vi "设置实验目录.vi"() -> ()   [LabVIEW 2013]
panel:
  in  "stop":bool
  in  "实验文件夹":path
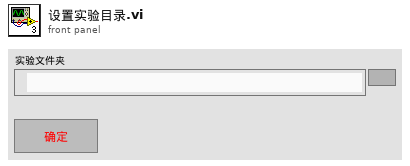
[diagram p1: front panel]
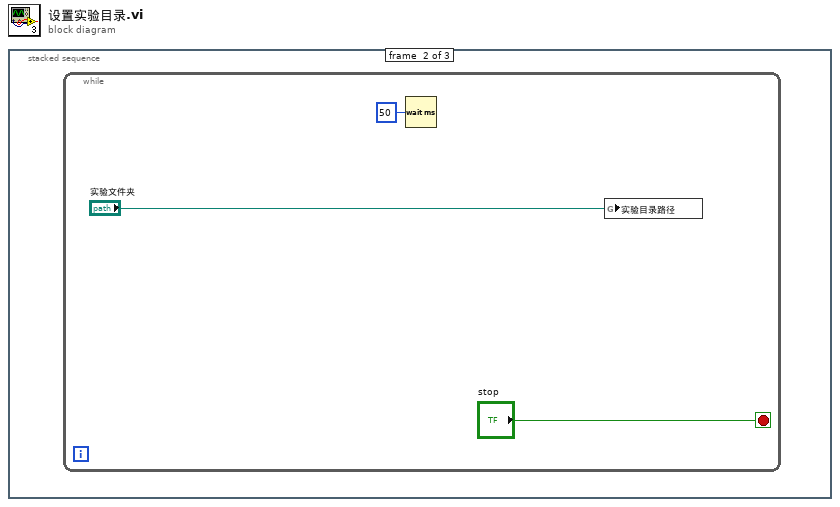
[diagram p0: block diagram]
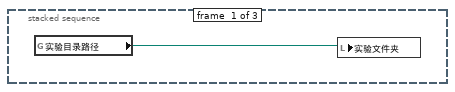
[diagram p2: hidden frame]
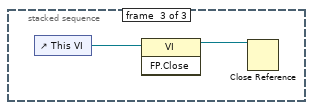
[diagram p3: hidden frame]
diagram:
  n1 = stacked-sequence {
    frame #0 {
      n2 = global read "实验目录路径.vi" "实验目录路径"() -> (w1:path)
      n3 = local write "实验文件夹"(w1) -> ()
    }
    frame #1 {
      n4 = while {
        stop <- "stop" stop-if-true
        n5 = Wait (ms)(milliseconds to wait=u32 50) -> ()  [unwired: 1 out]
        n6 = global write "实验目录路径.vi" "实验目录路径"("实验文件夹") -> ()
      }
    }
    frame #2 {
      n7 = control-ref of="This VI"() -> (w6:refnum<vi>)
      n8 = invoke class="VI" method="FP.Close"(reference=w6) -> (reference out=w5:refnum<vi>)  [unwired: 2 in, 2 out]
      n9 = Close Reference(reference=w5) -> ()  [unwired: 1 in, 1 out]
    }
  }
